vi "Ohaus Scout (com5).vi"(4 "State":i16, 5 "Time":dbl format="%.2f", 6 "Sensor Values":dbl[](array[numeric]), 7 "Set Points":dbl[](array[numeric])) -> (0 "required data":T1, 3 "output value":dbl)   [LabVIEW 2019]
uses:
  <vilib>/Instr/_visa.llb/VISA Configure Serial Port (Instr).vi
panel:
  in  "String":string
  out "write buffer":string
  out "VISA resource name out":refnum<visa-resource-name>
  # "Enter the correct information for this control code in the required data structure below. Then make the current value default by right clicking on the border of the data structure. Select \"data operations\" and then select \"make current value default\". These values will be displayed by process controller."
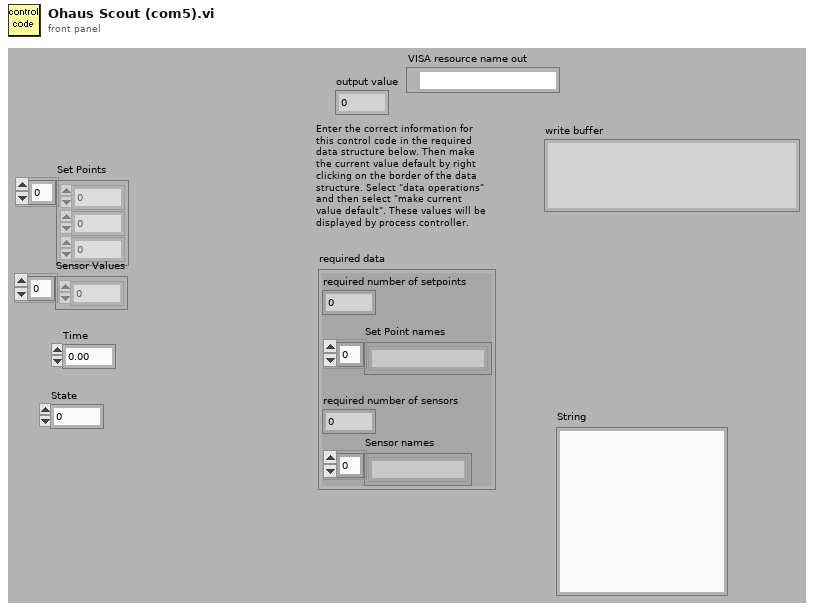
[diagram p1: front panel]
types:
  T1 = cluster{"Set Point names":string[], "required number of setpoints":u8, "required number of sensors":u8, "Sensor names":string[]}
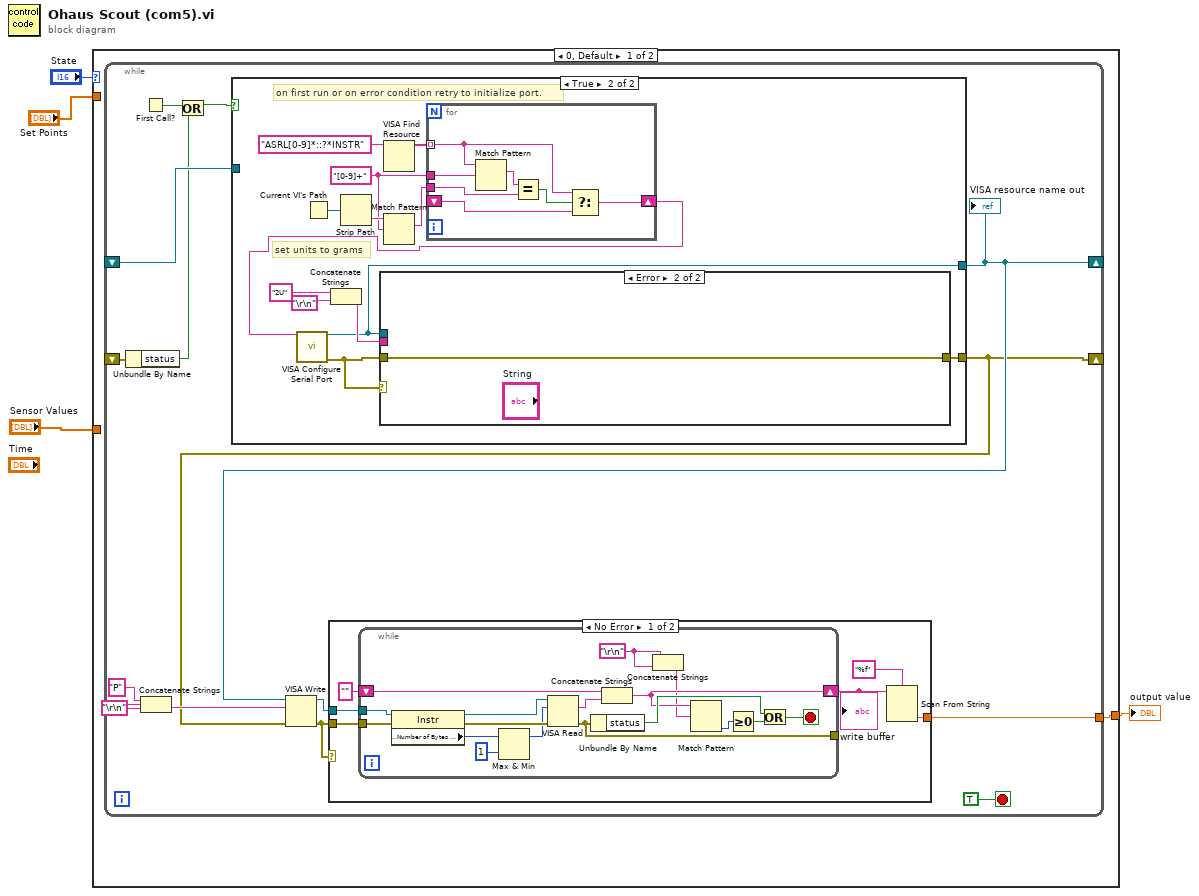
[diagram p0: block diagram]
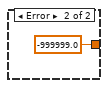
[diagram p2: hidden frame]
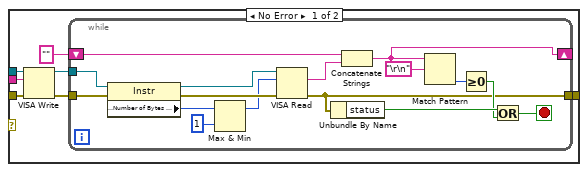
[diagram p4: hidden frame]
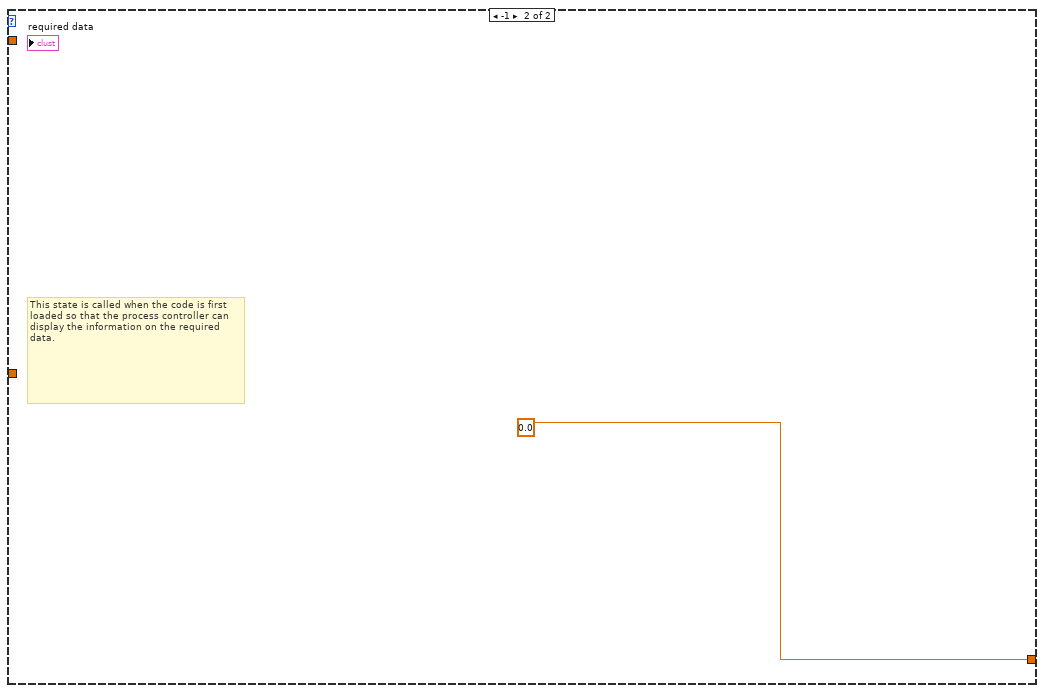
[diagram p5: hidden frame]
diagram:
  n1 = case shown="0, Default" "State" {
    tunnel: [w5 0.0 ("fraction on")] -> w3
    tunnel: "Set Points" -> [_ _]
    tunnel: "Sensor Values" -> [_ _]
    frame 0, Default {
      n2 = while {
        tunnel: [w19] -> w5
        shift-right: [w12] -> _
        shift-left: _ -> [w13]
        shift-right: [w10] -> _
        shift-left: _ -> [w9]
        stop <- TRUE stop-if-true
        n3 = Unbundle By Name(w9) -> ("status"=w7:bool)
        n4 = First Call?() -> (First Call?: T/F=w17:bool)
        n5 = Concatenate Strings("P", "\r\n") -> (w14:string)
        n6 = Or(x=w17, y=w7) -> (x .or. y?=w8:bool)
        n7 = case shown="True" w8 {
          tunnel: [_ w54] -> w10
          tunnel: [w44 w46] -> w12
          tunnel: w13 -> [w44 _]
          frame False {
          }
          frame True {
            w48 = "[0-9]+" ("regular expression")
            # "on first run or on error condition retry to initialize port."
            # "set units to grams"
            n8 = Current VI's Path() -> (path=w53:path)
            n9 = Concatenate Strings("2U", "\r\n") -> (w55:string)
            n10 = Strip Path(path=w53) -> (name=w52:string)  [unwired: 1 out]
            n11 = VISA Find Resource(11:"ASRL[0-9]*::?*INSTR" ("expression (\"?*\")")) -> (3:w50:string[])  [unwired: 2 in, 2 out]
            n12 = Match Pattern(string=w52, regular expression=w48) -> (match substring=w49:string)  [unwired: 1 in, 3 out]
            n13 = for {
              tunnel: w50 -> [w83] mode=indexing
              tunnel: w49 -> [w87]
              shift-right: [w84] -> w47
              shift-left: _ -> [w85]
              tunnel: w48 -> [w82]
              n14 = Match Pattern(string=w83, regular expression=w82) -> (match substring=w88:string)  [unwired: 1 in, 3 out]
              n15 = Equal?(x=w88, y=w87) -> (x = y?=w86:bool)
              n16 = Select(t=w83, s=w86, f=w85) -> (s? t:f=w84:string)
            }
            n17 = call-poly "VISA Configure Serial Port"("VISA resource name"=w47) -> ("VISA resource name out"=w46:refnum<visa-resource-name>, "error out"=w45:errorcluster)  [unwired: 13 in]
            n18 = case shown="Error" w45 {
              tunnel: w55 -> [w62 _]
              tunnel: w45 -> [w61 w81]
              tunnel: [w59 w81] -> w54
              tunnel: w46 -> [w58 _]
              frame No Error {
                n19 = VISA Write(VISA resource name=w58, write buffer=w62, error in (no error)=w61) -> (VISA resource name out=w60:refnum<visa-resource-name>, error out=w64:errorcluster)  [unwired: 1 out]
                n20 = while {
                  tunnel: w60 -> [w79]
                  tunnel: w64 -> [w77]
                  shift-right: [w65] -> _
                  shift-left: "" ("write buffer") -> [w80]
                  tunnel: [w66] -> w59
                  stop <- w75 stop-if-true
                  n21 = property class="Instr"(reference=w79, error in=w77) -> (reference out=w78:refnum<visa-resource-name>, error out=w76:errorcluster, "Serial Settings:Number of Bytes at Serial Port"=w68:u32)
                  n22 = Max & Min(x=w68, y=u32 1) -> (max(x,y)=w69:u32)  [unwired: 1 out]
                  n23 = VISA Read(VISA resource name=w78, byte count=w69, error in (no error)=w76) -> (read buffer=w73:string, error out=w66:errorcluster)  [unwired: 2 out]
                  n24 = Unbundle By Name(w66) -> ("status"=w74:bool)
                  n25 = Concatenate Strings(w80, w73) -> (w65:string)
                  n26 = Match Pattern(string=w65, regular expression="\r\n") -> (offset past match=w71:i32)  [unwired: 1 in, 3 out]
                  n27 = Greater Or Equal To 0?(x=w71) -> (x >= 0?=w70:bool)
                  n28 = Or(x=w74, y=w70) -> (x .or. y?=w75:bool)
                }
              }
              frame Error {
              }
            }
          }
        }
        "VISA resource name out" <- w12
        n29 = VISA Write(VISA resource name=w12, write buffer=w14, error in (no error)=w10) -> (VISA resource name out=w18:refnum<visa-resource-name>, error out=w6:errorcluster)  [unwired: 1 out]
        n30 = case shown="No Error" w6 {
          tunnel: [w25 -999999.0] -> w19
          tunnel: w18 -> [w24 _]
          tunnel: w6 -> [w23 _]
          frame No Error {
            n31 = while {
              tunnel: w24 -> [w41]
              tunnel: w23 -> [w39]
              shift-right: [w29] -> w20
              shift-left: "" ("write buffer") -> [w42]
              tunnel: [w30] -> _
              stop <- w37 stop-if-true
              w27 = "\r\n"
              n32 = property class="Instr"(reference=w41, error in=w39) -> (reference out=w40:refnum<visa-resource-name>, error out=w38:errorcluster, "Serial Settings:Number of Bytes at Serial Port"=w32:u32)
              n33 = Max & Min(x=w32, y=u32 1) -> (max(x,y)=w33:u32)  [unwired: 1 out]
              n34 = VISA Read(VISA resource name=w40, byte count=w33, error in (no error)=w38) -> (read buffer=w35:string, error out=w30:errorcluster)  [unwired: 2 out]
              n35 = Unbundle By Name(w30) -> ("status"=w36:bool)
              n36 = Concatenate Strings(w42, w35) -> (w29:string)
              n37 = Concatenate Strings(w27, w27) -> (w28:string)
              n38 = Match Pattern(string=w29, regular expression=w28) -> (offset past match=w34:i32)  [unwired: 1 in, 3 out]
              n39 = Greater Or Equal To 0?(x=w34) -> (x >= 0?=w26:bool)
              n40 = Or(x=w36, y=w26) -> (x .or. y?=w37:bool)
            }
            "write buffer" <- w20
            n41 = Scan From String(format string="%f", input string=w20) -> (output 1=w25:dbl)  [unwired: 3 in, 3 out]
          }
          frame Error {
          }
        }
      }
    }
    frame -1 {
      # "This state is called when the code is first loaded so that the process controller can display the information on the required data."
    }
  }
  "output value" <- w3
